vi "exp8 structures.vi"() -> ()   [LabVIEW 2025]
panel:
  in  "message":string
  in  "Boolean 8":bool
  out "Boolean 4":bool
  out "Boolean 3":bool
  out "Boolean 2":bool
  in  "stop 2":bool
  in  "mul":bool
  in  "add":bool
  out "Numeric":i32
  in  "stop":bool
  in  "Boolean":bool
  out "x+y":i32
  # "case: to make decisions"
  # "event"
  # "flat sequence"
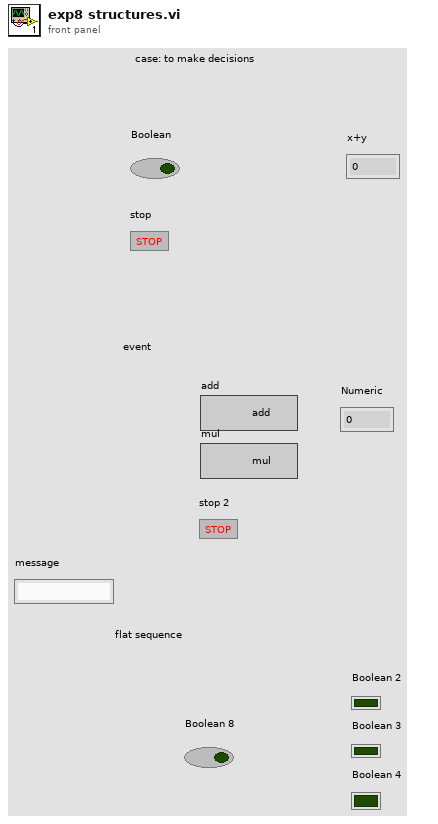
[diagram p1: front panel]
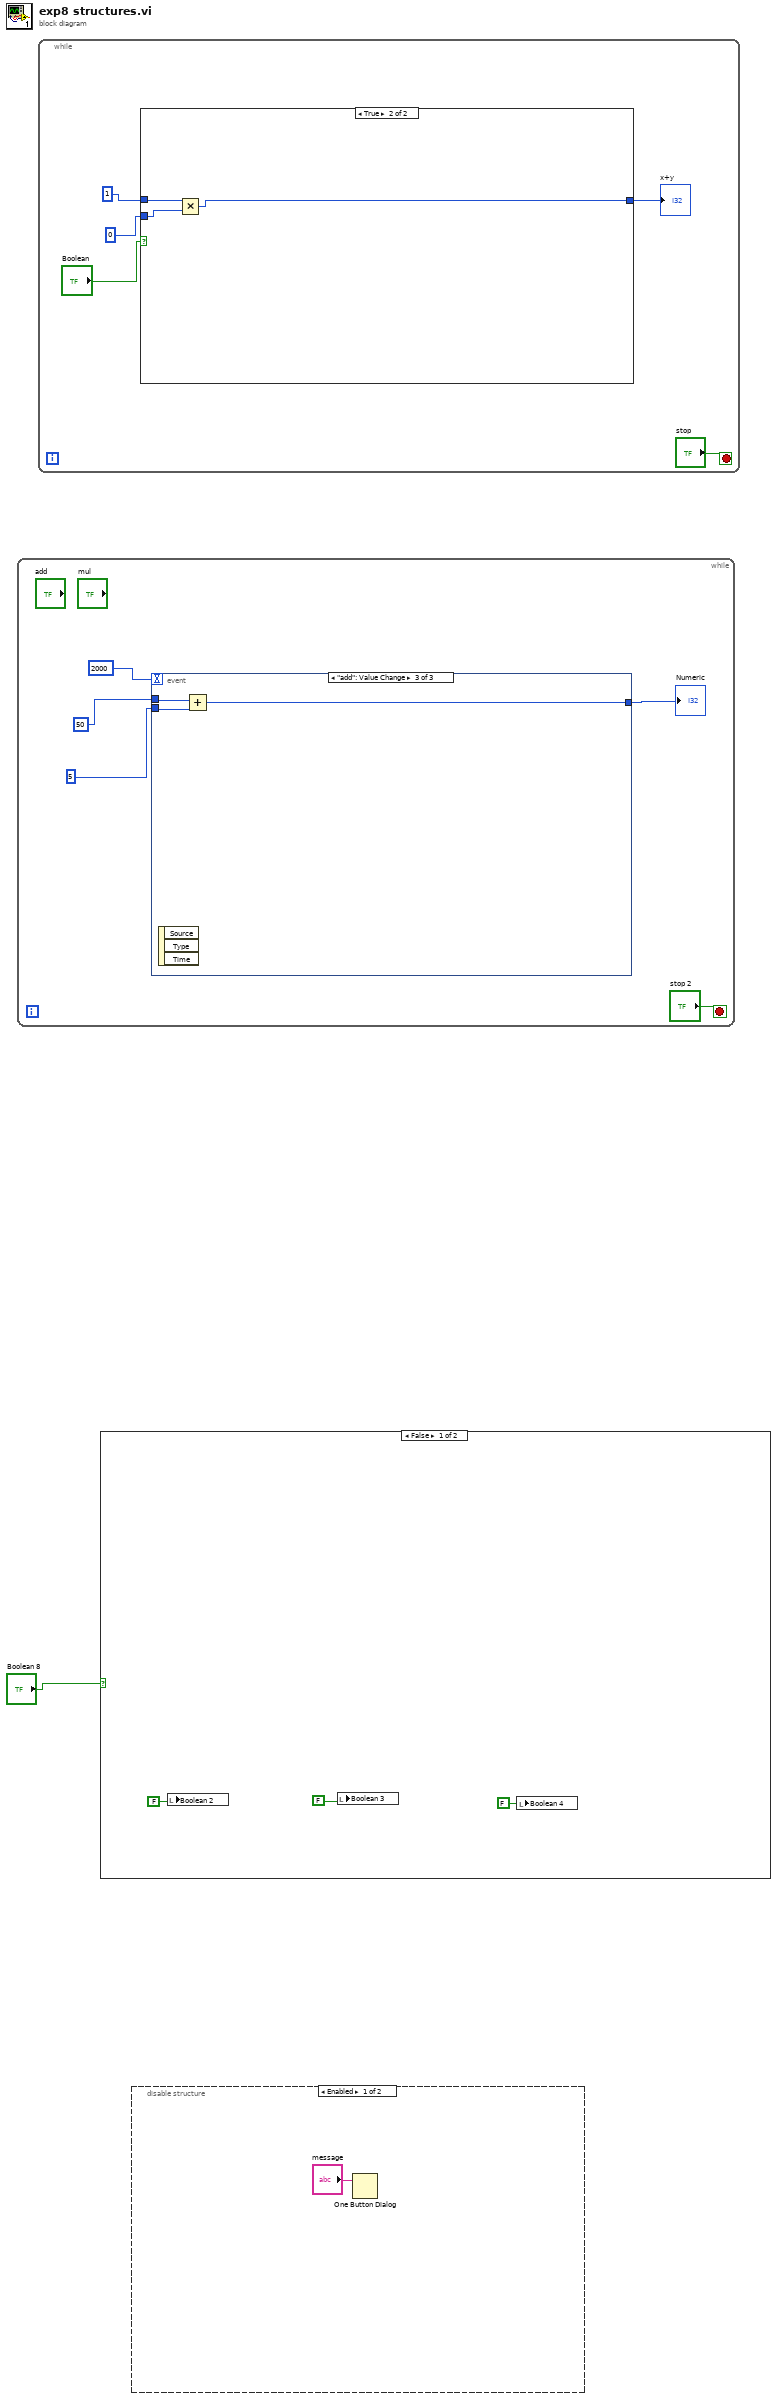
[diagram p0: block diagram]
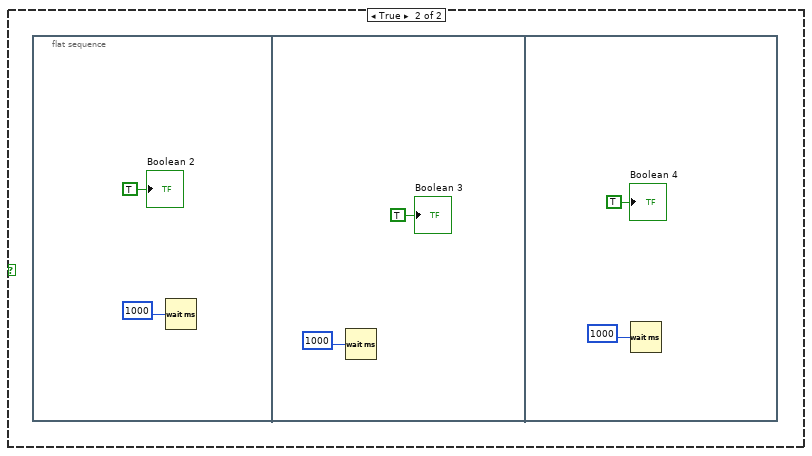
[diagram p3: hidden frame]
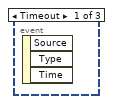
[diagram p4: hidden frame]
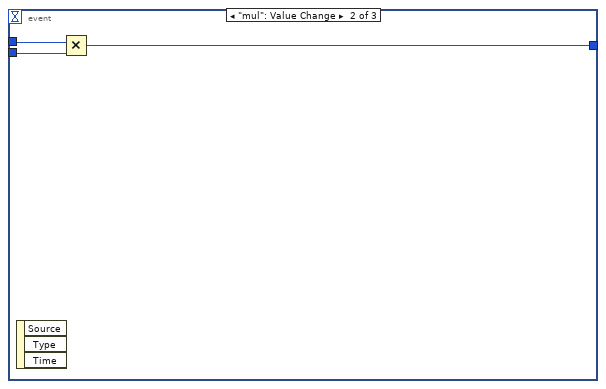
[diagram p5: hidden frame]
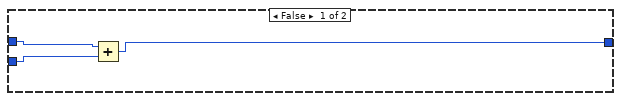
[diagram p6: hidden frame]
diagram:
  n1 = while {
    stop <- "stop 2" stop-if-true
    n2 = event shown="[2] \"add\": Value Change" {
      selector: _ -> [_ _ _]
      dyn-events: _ -> [_ _ _]
      timeout: 2000 ("Numeric 2") -> [_ _ _]
      tunnel: 50 -> [_ w9 w12]
      tunnel: 5 -> [_ w8 w11]
      tunnel: [_ w7 w10] -> w4
      event Timeout {
        n3 = event-data() -> ()  [unwired: 1 in, 3 out]
      }
      event "mul": Value Change {
        n4 = event-data() -> ()  [unwired: 1 in, 3 out]
        n5 = Multiply(x=w9, y=w8) -> (x*y=w7:i32)
      }
      event "add": Value Change {
        n6 = event-data() -> ()  [unwired: 1 in, 3 out]
        n7 = Add(x=w12, y=w11) -> (x+y=w10:i32)
      }
    }
    "Numeric" <- w4
  }
  n8 = while {
    stop <- "stop" stop-if-true
    n9 = case shown="True" "Boolean" {
      tunnel: 0 -> [w19 w22]
      tunnel: 1 -> [w20 w23]
      tunnel: [w18 w21] -> w15
      frame False {
        n10 = Add(x=w20, y=w19) -> (x+y=w18:i32)
      }
      frame True {
        n11 = Multiply(x=w23, y=w22) -> (x*y=w21:i32)
      }
    }
    "x+y" <- w15
  }
  n12 = case shown="False" "Boolean 8" {
    frame False {
      n13 = local write "Boolean 2"(FALSE ("Boolean 2")) -> ()
      n14 = local write "Boolean 3"(FALSE ("Boolean 3")) -> ()
      n15 = local write "Boolean 4"(FALSE ("Boolean 4")) -> ()
    }
    frame True {
      n16 = flat-sequence {
        frame #0 {
          n17 = Wait (ms)(milliseconds to wait=1000) -> ()  [unwired: 1 out]
          "Boolean 2" <- TRUE ("Boolean 2")
        }
        frame #1 {
          n18 = Wait (ms)(milliseconds to wait=1000) -> ()  [unwired: 1 out]
          "Boolean 3" <- TRUE ("Boolean 2")
        }
        frame #2 {
          n19 = Wait (ms)(milliseconds to wait=1000) -> ()  [unwired: 1 out]
          "Boolean 4" <- TRUE ("Boolean 2")
        }
      }
    }
  }
  n20 = disable-structure shown="Enabled" {
    frame Enabled {
      n21 = One Button Dialog(message="message") -> ()  [unwired: 1 in, 1 out]
    }
    frame Disabled {
    }
  }
